vi "CT-Sweep Amplitude.vi"(0 "Y In":dbl[](array[numeric]), 5 "Astart":dbl=2000.0, 7 "Aend":dbl=2000.0, 11 "Npts":i32) -> (4 "Y Out":dbl[](array[numeric]))   [LabVIEW 2015]
uses:
  Utility VIs/Math VIs/LinSpace (x0-dx-npts).vi
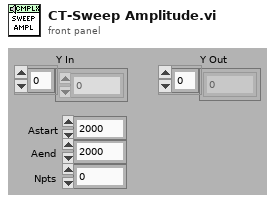
[diagram p1: front panel]
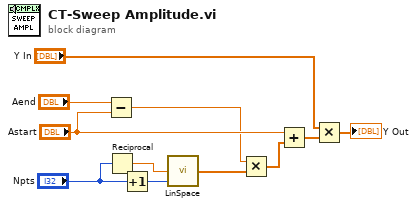
[diagram p0: block diagram]
diagram:
  n1 = Subtract(x="Aend", y="Astart") -> (x-y=w9:dbl)
  n2 = Reciprocal(x="Npts") -> (1/x=w1:dbl)
  n3 = Increment(x="Npts") -> (x+1=w4:i32)
  n4 = call-poly "LinSpace.vi"("npts"=w4, "dx"=w1) -> ("Array"=w3:dbl[])  [unwired: 2 in, 1 out]
  n5 = Multiply(x=w9, y=w3) -> (x*y=w8:dbl[])
  n6 = Add(x="Astart", y=w8) -> (x+y=w7:dbl[])
  n7 = Multiply(x="Y In", y=w7) -> (x*y=→"Y Out":dbl[])
